vi "Read Ch2Delay.vi"(8 "error in (no error)":errorcluster, 11 "Pulse Generator in":refnum<class "Pulse Generator.lvclass">) -> (0 "error out":errorcluster, 2 "Ch2Delay":dbl[unit], 3 "Pulse Generator out":refnum<class "Pulse Generator.lvclass">)   [LabVIEW 2017, in "Pulse Generator.lvclass"]
uses:
  Pulse Generator.lvclass
  Pulse Generator.lvclass/Pulse Generator.ctl
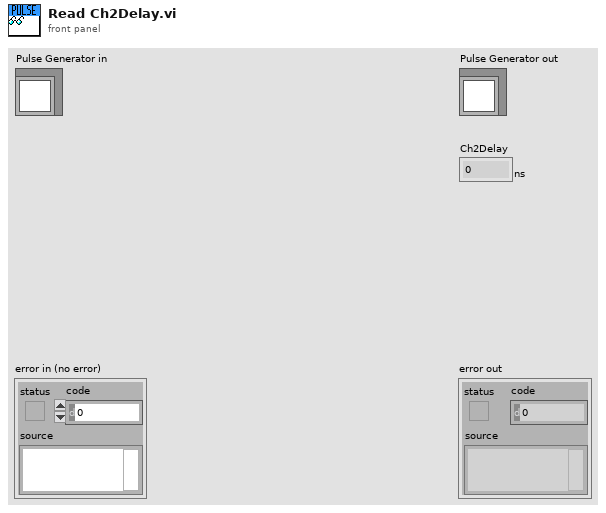
[diagram p1: front panel]
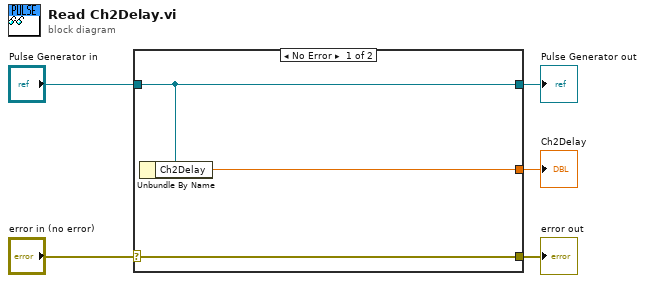
[diagram p0: block diagram]
diagram:
  n1 = case shown="No Error" "error in (no error)" {
    selector: "error in (no error)" -> [w8 w9]
    tunnel: [w8 w9] -> w4
    tunnel: [w7 w10] -> w2
    tunnel: "Pulse Generator in" -> [w7 w10]
    tunnel: [w6 _] -> w1
    frame No Error {
      n2 = Unbundle By Name(w7) -> ("Ch2Delay"=w6:dbl[unit])
    }
    frame Error {
    }
  }
  "error out" <- w4
  "Pulse Generator out" <- w2
  "Ch2Delay" <- w1
